vi "apply data indices.vi"(8 "error in":errorcluster, 10 "index type defs":T1, 11 "fixed channel tag bus module in":refnum<class "fixed channel tag bus module.lvclass">) -> (0 "error out":errorcluster, 3 "fixed channel tag bus module out":refnum<class "fixed channel tag bus module.lvclass">)   [LabVIEW 2013, in "fixed channel tag bus module.lvclass"]
uses:
  fixed channel tag bus module.lvclass
  fixed module parent/module/configuration/index type definitions.ctl
  configuration/input data indices.ctl
  configuration/output data indices.ctl
  configuration/parameter data indices.ctl
  configuration/result data indices.ctl
  fixed channel tag bus module.lvclass/fixed channel tag bus module.ctl
  configuration/fixed channel tag bus module configuration.lvclass
  fixed module parent/module/configuration/fixed channel configuration.lvclass
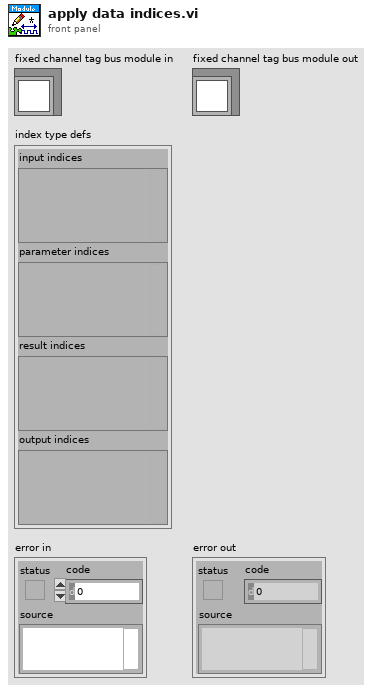
[diagram p1: front panel]
types:
  T1 = typedef "fixed channel configuration.lvclass/index type definitions.ctl" = cluster{"input indices":variant, "parameter indices":variant, "result indices":variant, "output indices":variant}
  T2 = typedef "fixed channel tag bus module configuration.lvclass/result data indices.ctl" = cluster{"Single.placeholder":i32}
  T3 = typedef "fixed channel tag bus module configuration.lvclass/parameter data indices.ctl" = cluster{"Single.placeholder":i32}
  T4 = typedef "fixed channel tag bus module configuration.lvclass/output data indices.ctl" = cluster{"Single.placeholder":i32}
  T5 = typedef "fixed channel tag bus module configuration.lvclass/input data indices.ctl" = cluster{"Single.placeholder":i32}
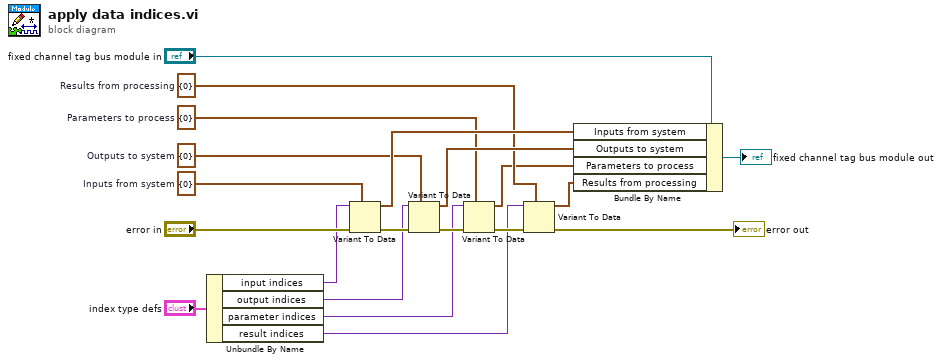
[diagram p0: block diagram]
diagram:
  w3 = T2 {"Single.placeholder"=0}  # Results from processing
  w4 = T3 {"Single.placeholder"=0}  # Parameters to process
  w8 = T4 {"Single.placeholder"=0}  # Outputs to system
  w11 = T5 {"Single.placeholder"=0}  # Inputs from system
  n1 = Unbundle By Name("index type defs") -> ("input indices"=w12:variant, "output indices"=w9:variant, "parameter indices"=w6:variant, "result indices"=w5:variant)
  n2 = Variant To Data(error in="error in", type=w11, Variant=w12) -> (data=w10:T5, error out=w13:errorcluster)
  n3 = Variant To Data(error in=w13, type=w8, Variant=w9) -> (data=w7:T4, error out=w16:errorcluster)
  n4 = Variant To Data(error in=w16, type=w4, Variant=w6) -> (data=w2:T3, error out=w14:errorcluster)
  n5 = Variant To Data(error in=w14, type=w3, Variant=w5) -> (data=w1:T2, error out=→"error out":errorcluster)
  n6 = Bundle By Name(cluster="fixed channel tag bus module in", "Inputs from system"=w10, "Outputs to system"=w7, "Parameters to process"=w2, "Results from processing"=w1) -> (→"fixed channel tag bus module out":refnum<class "fixed channel tag bus module.lvclass">)
